vi "para1.vi"(4 "User Parameter":variant, 5 "Event Data":T2, 6 "Control Ref":refnum<k7>, 7 "Event Common Data":T3) -> (1 "Event Data Out":T1)   [LabVIEW 2012]
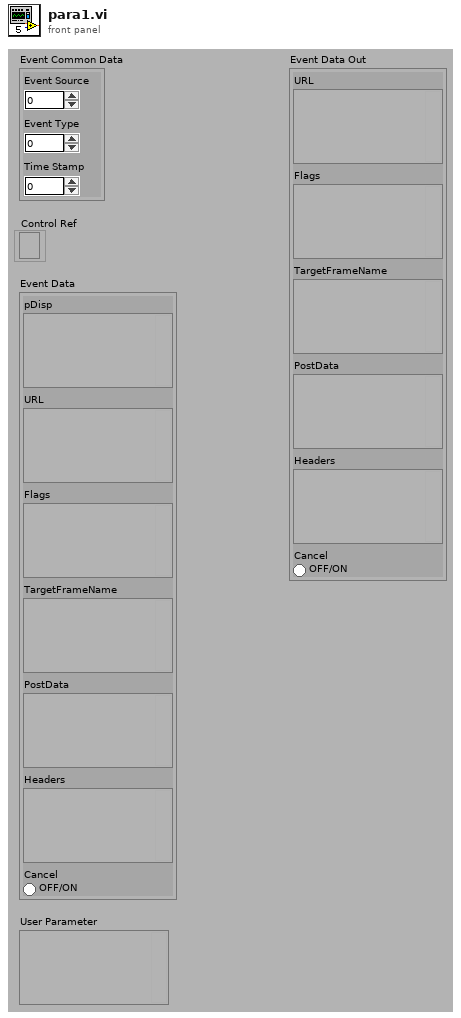
[diagram p1: front panel]
types:
  T1 = cluster{"URL":variant, "Flags":variant, "TargetFrameName":variant, "PostData":variant, "Headers":variant, "Cancel":bool}
  T2 = cluster{"pDisp":variant, "URL":variant, "Flags":variant, "TargetFrameName":variant, "PostData":variant, "Headers":variant, "Cancel":bool}
  T3 = cluster{"Event Source":i32, "Event Type":u32, "Time Stamp":u32}
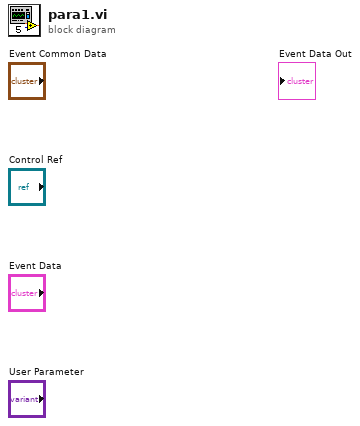
[diagram p0: block diagram]
diagram:
